vi "Host_UDPLoop.vi"(8 "error in (no error)":errorcluster) -> (0 "error out":errorcluster)   [LabVIEW 2017]
doc: "Contains the loop for formatting and sending UDP messages according to SpaceX's requirements:\npackage must include:\nUINT8 team_id\nUINT8 Status\nINT32 Acceleration cm2/s\nINT32 Position cm\nINT32 Velocity cm/s\nINT32 battery_voltage mV\nINT32 battery_current mA\nINT32 battery_temperature tenths of C\nINT32 pod_temperature tenths of C\nUINT32 Stripe count"
uses:
  Globals/Host_UDPGLOBALS.vi
  Globals/Host_STOP.vi
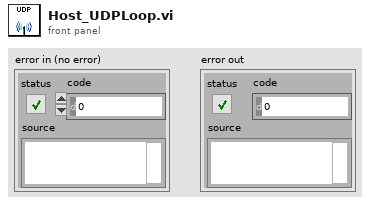
[diagram p1: front panel]
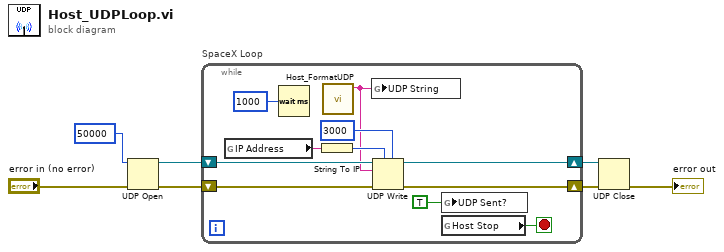
[diagram p0: block diagram]
diagram:
  n1 = UDP Open(8:"error in (no error)", 11:u16 50000 ("port")) -> (port=w3:refnum<k16>, 0:w4:errorcluster)  [unwired: 3 in, 1 out]
  n2 = while "SpaceX Loop" {
    shift-right: [w18] -> w1
    shift-left: w3 -> [w17]
    shift-right: [w9] -> w2
    shift-left: w4 -> [w12]
    stop <- w13 stop-if-true
    n3 = global read "Host_UDPGLOBALS.vi" "IP Address"() -> (w11:string)
    n4 = Wait (ms)(milliseconds to wait=u32 1000) -> ()  [unwired: 1 out]
    n5 = String To IP(1:w11) -> (0:w15:u32)
    n6 = call "Host_FormatUDP.vi"() -> ("data string"=w10:string)  [unwired: 11 in]
    n7 = global write "Host_UDPGLOBALS.vi" "UDP String"(w10) -> ()
    n8 = UDP Write(address=w15, port or service name=u16 3000, connection ID=w17, data in=w10, 8:w12) -> (error out=w9:errorcluster, 3:w18:refnum<k16>)  [unwired: 1 in]
    n9 = global write "Host_UDPGLOBALS.vi" "UDP Sent?"(TRUE) -> ()
    n10 = global read "Host_STOP.vi" "Host Stop"() -> (w13:bool)
  }
  n11 = UDP Close(connection ID=w1, 8:w2) -> (error out=→"error out":errorcluster)  [unwired: 1 out]
